vi "_Destroy.vi"(8 "Error In":errorcluster, 11 "Log In":refnum<file>) -> (0 "Error Out":errorcluster, 3 "Base Log Folder":path)   [LabVIEW 2014, in "CF-Logger.lvlib"]
uses:
  CF-Logger.lvlib
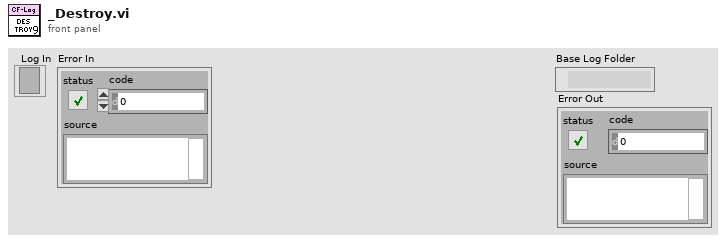
[diagram p1: front panel]
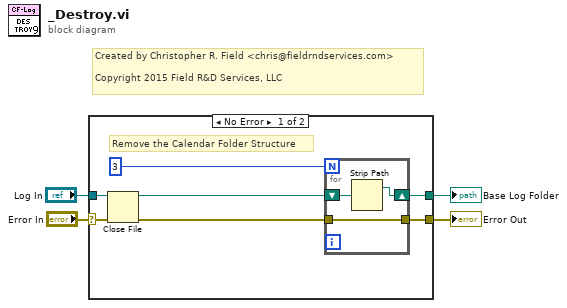
[diagram p0: block diagram]
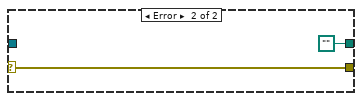
[diagram p2: hidden frame]
diagram:
  # "Created by Christopher R. Field <chris@fieldrndservices.com>\n\nCopyright 2015 Field R&D Services, LLC"
  n1 = case shown="No Error" "Error In" {
    selector: "Error In" -> [w10 w16]
    tunnel: "Log In" -> [w11 _]
    tunnel: [w6 path ""] -> w2
    tunnel: [w5 w16] -> w1
    frame No Error {
      # "Remove the Calendar Folder Structure"
      n2 = Close File(refnum=w11, error in=w10) -> (path=w9:path, error out=w8:errorcluster)
      n3 = for {
        N: 3 -> [_]
        shift-right: [w13] -> w6
        shift-left: w9 -> [w14]
        tunnel: w8 -> [w12]
        tunnel: [w12] -> w5
        n4 = Strip Path(path=w14) -> (stripped path=w13:path)  [unwired: 1 out]
      }
    }
    frame Error {
    }
  }
  "Base Log Folder" <- w2
  "Error Out" <- w1
